vi "Show Fs.vi"(0 "Display State In":T1, 5 "Show":bool, 9 "Container State":T5, 11 "error in (no error)":errorcluster) -> (4 "Display State Out":T1, 15 "error out":errorcluster)   [LabVIEW 2015, in "SignalManager.xctl"]
uses:
  SignalManager.xctl
  <vilib>/_xctls/Container State.ctl
  State.ctl
  Utility VIs/Controls/KListboxEx/Events.ctl
  Utility VIs/Controls/KListboxEx/Event Action.ctl
  PeriodDisplay.ctl
  Events.ctl
  Event Data.ctl
  <vilib>/_xctls/XControlSupport.lvlib
  Utility VIs/Controls/KListboxEx/KListboxEx.xctl
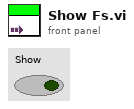
[diagram p1: front panel]
types:
  T1 = typedef "SignalManager.xctl/State.ctl" = cluster{"Channels":T2, "Destinations":string[], "action":string, "EventReg":refnum<event-registration>, "selectedChan":i32, "Period Display":T3, "Events":T4}
  T2 = typedef "KListboxEx.xctl/Events.ctl" = cluster{"Items Changed":refnum<user-event>, "List Changed":refnum<user-event>}
  T3 = typedef "SignalManager.xctl/PeriodDisplay.ctl" = enum16{"Interval", "RepRate", "Both"}
  T4 = typedef "SignalManager.xctl/Events.ctl" = cluster{"Rename":refnum<user-event>}
  T5 = typedef "XControlSupport.lvlib/Container State.ctl" = cluster{"Indicator?":bool, "Run Mode?":bool, " Refnum":refnum<vi>}
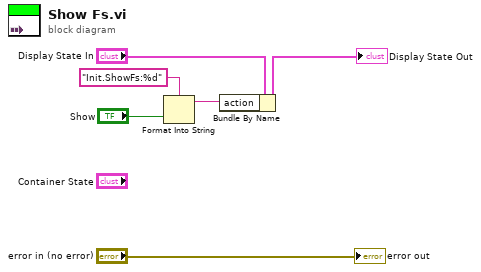
[diagram p0: block diagram]
diagram:
  n1 = Format Into String(format string="Init.ShowFs:%d", "Show") -> (resulting string=w1:string)  [unwired: 2 in, 1 out]
  n2 = Bundle By Name(cluster="Display State In", "action"=w1) -> (→"Display State Out":T1)
  "error out" <- "error in (no error)"
